vi "Config_32AI_Module_NI_0_10V.vi"(8 "error in (no error)":errorcluster, 10 "MODULE NAME":string, 11 "Refnum in":refnum<k21>) -> (0 "error out":errorcluster, 3 "Refnum out":refnum<k21>)   [LabVIEW 2019]
uses:
  <vilib>/DAQmx/create/channels.llb/DAQmx Create Channel (AI-Voltage-Basic).vi
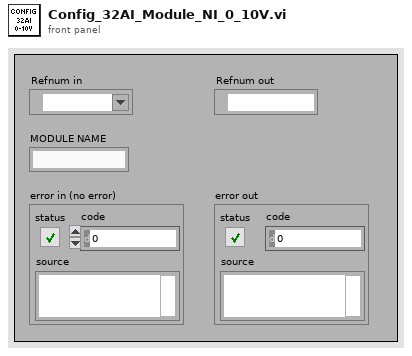
[diagram p1: front panel]
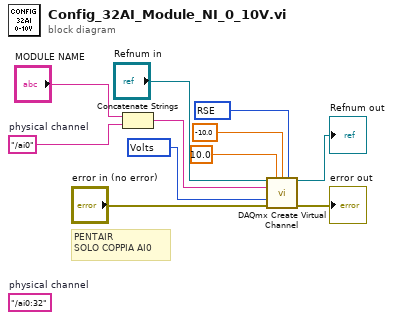
[diagram p0: block diagram]
diagram:
  (unwired) "/ai0:32"  # physical channel
  w1 = 10083 items=["Default"=-1, "RSE"=10083, "NRSE"=10078, "Differential"=10106, "Pseudodifferential"=12529] ("input terminal configuration")
  w6 = 10348 items=["Volts"=10348, "From Custom Scale"=10065] ("units")
  w9 = "/ai0"  # physical channel
  # "PENTAIR\nSOLO COPPIA AI0"
  n1 = Concatenate Strings("MODULE NAME", w9) -> (w10:string)
  n2 = call-poly <vilib>:"DAQmx Create Virtual Channel.vi"("task in"="Refnum in", "maximum value"=10.0, "minimum value"=-10.0, "input terminal configuration"=w1, "physical channels"=w10, "units"=w6, "error in"="error in (no error)") -> ("task out"=→"Refnum out":refnum<k21>, "error out"=→"error out":errorcluster)  [unwired: 7 in]
